vi "匹配NMEA字段.vi"(11 "输入字符串":string) -> (1 "未匹配语句":string, 2 "NMEA语句":string, 3 "匹配语句":string, 5 "匹配":bool)   [LabVIEW 2016, in "环境动力监测库.lvlib" / "AIRMAR WeatherCaster.lvlib"]
uses:
  AIRMAR WeatherCaster.lvlib
  <vilib>/regexp/Match Regular Expression.xnode
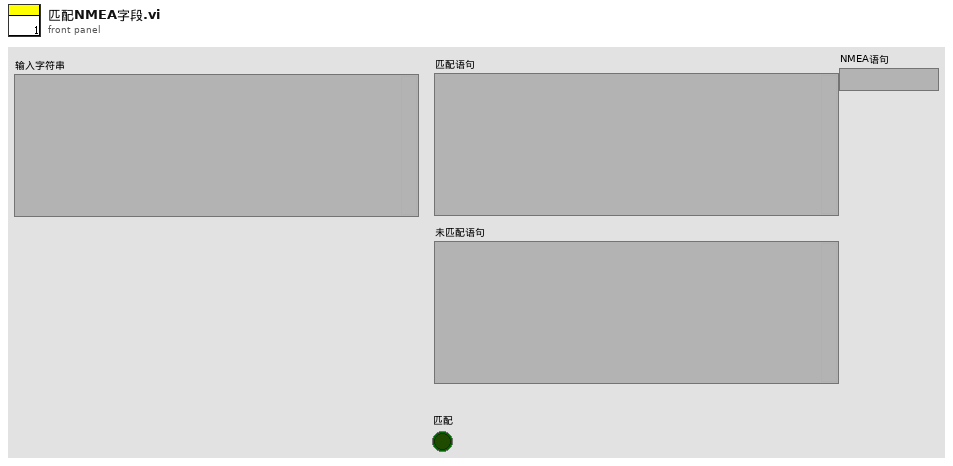
[diagram p1: front panel]
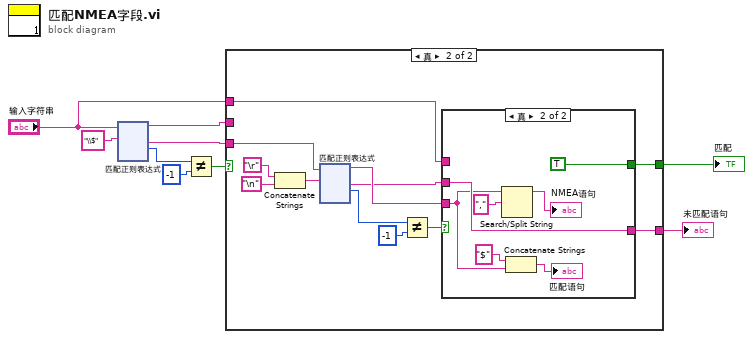
[diagram p0: block diagram]
diagram:
  n1 = xnode "匹配正则表达式"("输入字符串"="输入字符串", "正则表达式"="\\$") -> ("匹配之前"=w3:string, "匹配之后"=w8:string, "匹配后偏移量"=w6:i32)  [unwired: 4 in, 2 out]
  n2 = Not Equal?(x=w6, y=-1) -> (x != y?=w4:bool)
  n3 = case shown="真" w4 {
    tunnel: [w10 w15] -> w9
    tunnel: w8 -> [_ w12]
    tunnel: w3 -> [_ _]
    tunnel: [_ w13] -> w2
    tunnel: "输入字符串" -> [w10 w11]
    frame False {
    }
    frame True {
      n4 = Concatenate Strings("\r", "\n") -> (w22:string)
      n5 = xnode "匹配正则表达式"("输入字符串"=w12, "正则表达式"=w22) -> ("匹配之前"=w19:string, "匹配之后"=w14:string, "匹配后偏移量"=w18:i32)  [unwired: 4 in, 2 out]
      n6 = Not Equal?(x=w18, y=-1) -> (x != y?=w16:bool)
      n7 = case shown="真" w16 {
        tunnel: w19 -> [_ w26]
        tunnel: [w23 w30] -> w15
        tunnel: w14 -> [_ w30]
        tunnel: [_ TRUE] -> w13
        tunnel: w11 -> [w23 _]
        frame False {
        }
        frame True {
          n8 = Search/Split String(string=w26, search string/char (-)="," ("搜索字符串/字符(-)")) -> (substring before match=→"NMEA语句":string)  [unwired: 1 in, 2 out]
          n9 = Concatenate Strings("$" ("字符串"), w26) -> (→"匹配语句":string)
        }
      }
    }
  }
  "未匹配语句" <- w9
  "匹配" <- w2
